vi "HardwareInitialize.vi"(8 "Error In":errorcluster, 11 "Executable Configuration":T1) -> (0 "Error Out":errorcluster, 3 "Keithley 7001 Out":refnum<visa-resource-name>)   [LabVIEW 2012]
uses:
  ExecutableConfiguration.ctl
  libs/LV-Utilities/LV-Utilities.lvlib
  driver/Keithley-7001.lvlib
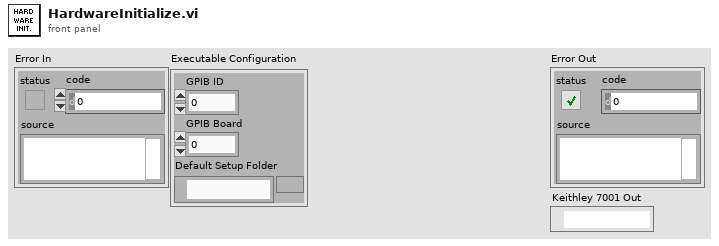
[diagram p1: front panel]
types:
  T1 = typedef "ExecutableConfiguration.ctl" = cluster{"GPIB ID":u8, "GPIB Board":u8, "Default Setup Folder":path}
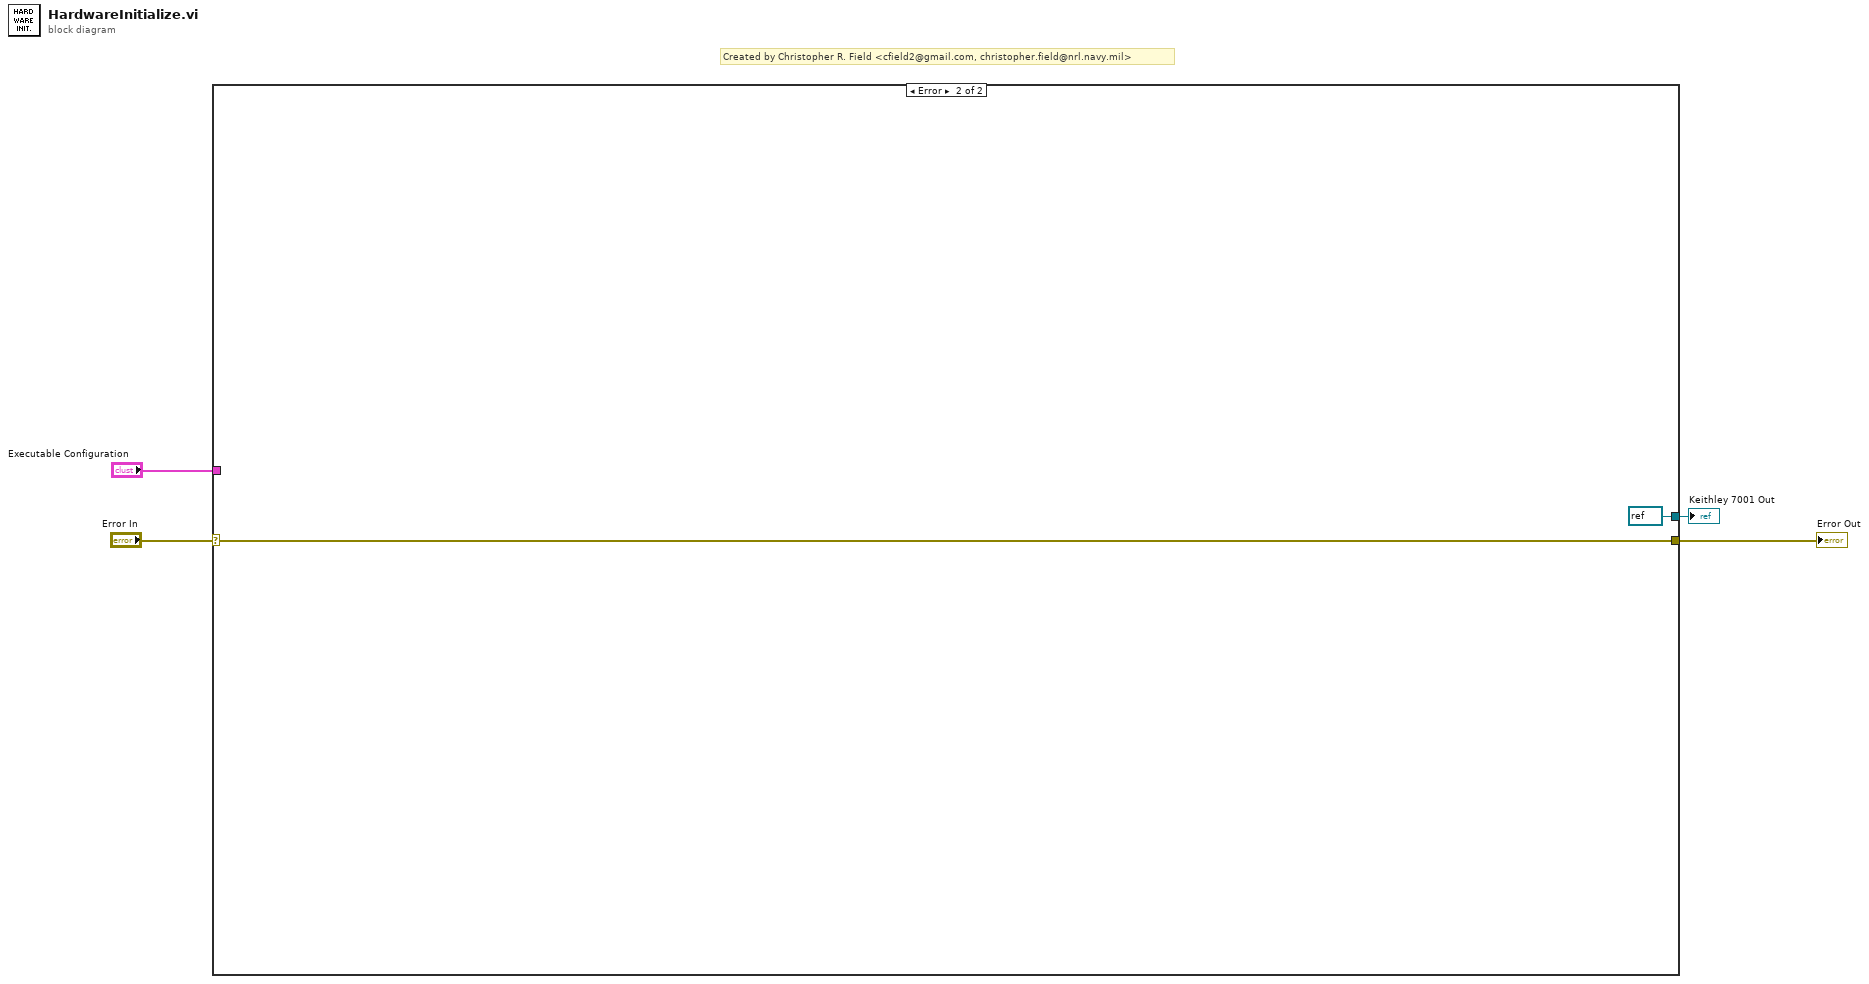
[diagram p0: block diagram]
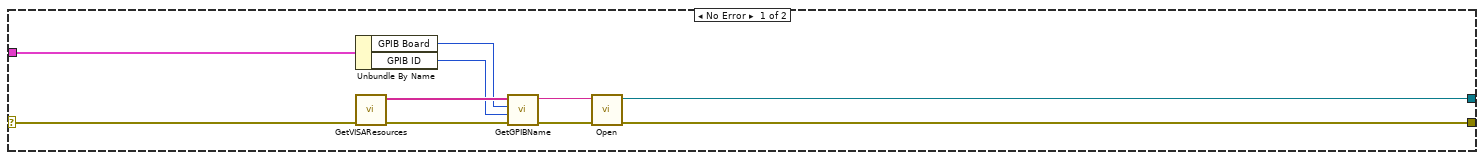
[diagram p2: hidden frame]
diagram:
  # "Created by Christopher R. Field <cfield2@gmail.com, christopher.field@nrl.navy.mil>"
  n1 = case shown="Error" "Error In" {
    selector: "Error In" -> [w8 w16]
    tunnel: "Executable Configuration" -> [w7 _]
    tunnel: [w6 w16] -> w2
    tunnel: [w5 refnum<visa-resource-name> refnum ("Keithley 7001 Out")] -> w1
    frame No Error {
      n2 = Unbundle By Name(w7) -> ("GPIB Board"=w12:u8, "GPIB ID"=w11:u8)
      n3 = call "GetVISAResources.vi"("Error In"=w8) -> ("Error Out"=w13:errorcluster, "VISA Resources"=w14:string[])  [unwired: 9 in]
      n4 = call "GetGPIBName.vi"("Error In"=w13, "GPIB ID"=w11, "GPIB Board"=w12, "VISA Resource List"=w14) -> ("Error Out"=w9:errorcluster, "VISA GPIB Resource Name"=w10:string)  [unwired: 5 in, 1 out]
      n5 = call "Open.vi"("Error In"=w9, "Keithley 7001 In"=w10) -> ("Error Out"=w6:errorcluster, "Keithley 7001 Out"=w5:refnum<visa-resource-name>)  [unwired: 8 in]
    }
    frame Error {
    }
  }
  "Error Out" <- w2
  "Keithley 7001 Out" <- w1
